vi "MLX Prog Flash.vi"(6 "nad":u8, 7 "AppFileName":string, 9 "LoaderFileName":string, 10 "LINChannel":u8, 11 "DeviceHandle":i32) -> (3 "function return":i32)   [LabVIEW 2010, in "mlx_programer.lvlib"]
doc: "int MLX_ProgFlash(int DeviceHandle, unsigned char LINChannel,const char* LoaderFileName,const char* AppFileName,unsigned char nad);"
uses:
  mlx_programer.lvlib
  USB2XXX/trunk/USB2XXX/USB2XXX/vs2010/Release/USB2XXX.dll
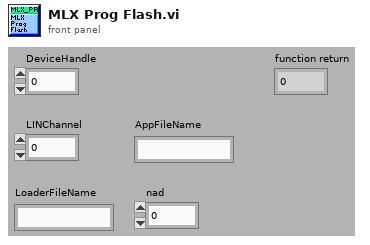
[diagram p1: front panel]
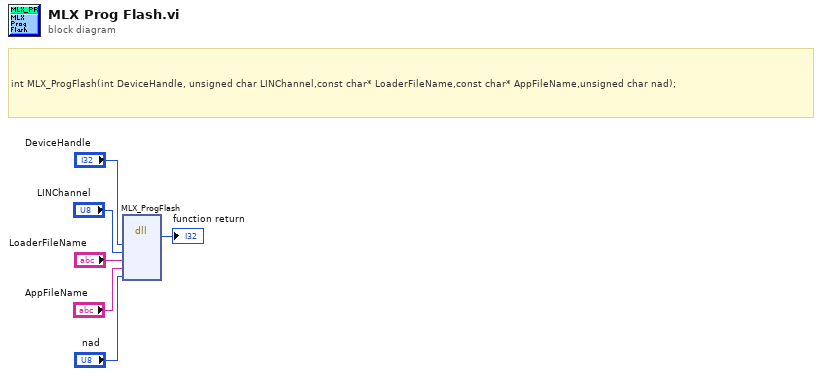
[diagram p0: block diagram]
diagram:
  # "int MLX_ProgFlash(int DeviceHandle, unsigned char LINChannel,const char* LoaderFileName,const char* AppFileName,unsigned char nad);"
  n1 = dll-call lib="E:/Projects/USB2XXX/trunk/USB2XXX/USB2XXX/vs2010/Release/USB2XXX.*" fn="MLX_ProgFlash"("DeviceHandle"="DeviceHandle", "LINChannel"="LINChannel", "LoaderFileName"="LoaderFileName", "AppFileName"="AppFileName", "nad"="nad") -> (→"function return":i32)  [unwired: 8 in, 2 out]
